vi "UI Loop Error and Que Setup.vi"(8 "error in (no error)":errorcluster, 11 "Receive Loop":refnum<user-event>) -> (0 "error out":errorcluster, 1 "UI Loop Event Registration":refnum<event-registration>, 2 "DAQ Queue":refnum<queue>, 3 "GEA Display Queue":refnum<queue>, 5 "ERD Queue Loop":refnum<queue>)   [LabVIEW 2023]
uses:
  type defs/ERD_Data_Loop_Control.ctl
  type defs/ERD_Loop_States.ctl
  GExplorer Support/typedefs/GExplorer_Data_Cluster.ctl
  type defs/DAQ_States.ctl
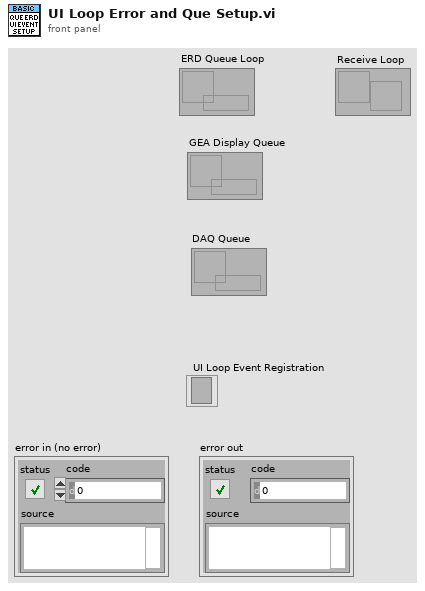
[diagram p1: front panel]
types:
  T1 = typedef "DAQ_States.ctl" = enum16{"Wait for Init", "Rename Devices", "Verify Hardware", "Initialize", "Run", "Shutdown", "Exit"}
  T2 = typedef "GExplorer_Data_Cluster.ctl" = cluster{"Data":variant, "State":enum16{"Add to Log", "Clear", "Shutdown"}}
  T3 = typedef "ERD_Data_Loop_Control.ctl" = cluster{"Data":variant, "State":T4}
  T4 = typedef "ERD_Loop_States.ctl" = enum16{"Init", "Build ERD Read List", "Read ERDs", "Get Version", "ERD´s User show", "Update UI", "Read Faults", "Log Data", "Pause", "Shutdown"}
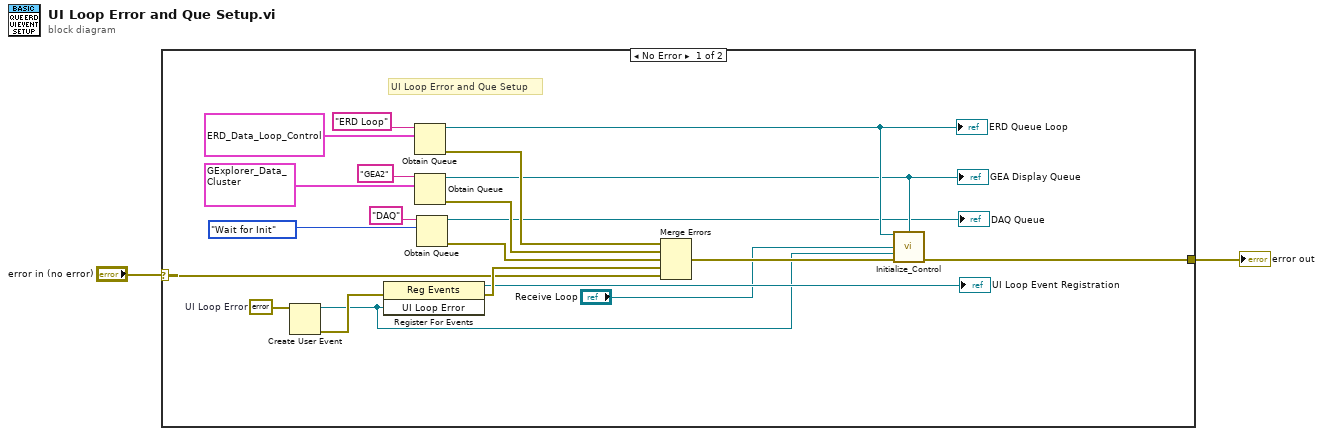
[diagram p0: block diagram]
diagram:
  n1 = case shown="No Error" "error in (no error)" {
    selector: "error in (no error)" -> [w10 w24]
    tunnel: [w23 w24] -> w2
    frame No Error {
      w15 = errorcluster {"status"=FALSE, "code"=0, "source"=""}  # UI Loop Error
      # "UI Loop Error and Que Setup"
      n2 = Create User Event(user event datatype=w15) -> (user event=w5:refnum<user-event>, error out=w16:errorcluster)  [unwired: 1 in]
      n3 = register-events(error in=w16, w5) -> (reference out=→"UI Loop Event Registration":refnum<event-registration>, error out=w11:errorcluster)  [unwired: 1 in]
      n4 = Obtain Queue(name (unnamed)="ERD Loop", element data type=T3 {"Data"=variant, "State"=enum."Read ERDs"} ("Data")) -> (queue out=w9:refnum<queue>, error out=w21:errorcluster)  [unwired: 3 in, 1 out]
      "ERD Queue Loop" <- w9
      n5 = Obtain Queue(name (unnamed)="GEA2", element data type=T2 {"Data"=variant, "State"=enum."Add to Log"} ("Data")) -> (queue out=w8:refnum<queue>, error out=w19:errorcluster)  [unwired: 3 in, 1 out]
      "GEA Display Queue" <- w8
      n6 = Obtain Queue(name (unnamed)="DAQ", element data type=DAQ_States."Wait for Init") -> (queue out=→"DAQ Queue":refnum<queue>, error out=w13:errorcluster)  [unwired: 3 in, 1 out]
      n7 = Merge Errors(w21, w19, w13, w11, w10) -> (w20:errorcluster)
      n8 = call "Initialize_Control.vi"("ERD Loop"=w9, "GEA2"=w8, "Receive Loop"="Receive Loop", "UI Loop Error"=w5, "Error In"=w20) -> ("Error Out"=w23:errorcluster)  [unwired: 10 in]
    }
    frame Error {
    }
  }
  "error out" <- w2
